vi "Complex Vector.vi"() -> (0 "error out":errorcluster, 3 "Passed?":bool)   [LabVIEW 2009]
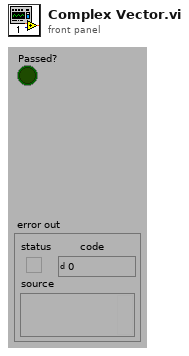
[diagram p1: front panel]
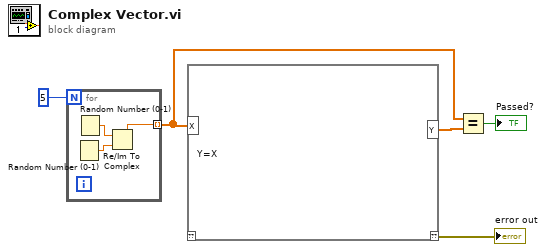
[diagram p0: block diagram]
diagram:
  n1 = for {
    N: 5 -> [_]
    tunnel: [w6] -> w2 mode=indexing
    n2 = Random Number (0-1)() -> (number: 0 to 1=w8:dbl)
    n3 = Random Number (0-1)() -> (number: 0 to 1=w7:dbl)
    n4 = Re/Im To Complex(1:w8, 2:w7) -> (0:w6:cdb)
  }
  n5 = script code="Y=X"("X"=w2) -> ("??"=→"error out":errorcluster, "Y"=w1:cdb[])  [unwired: 1 in]
  n6 = Equal?(x=w2, y=w1) -> (x = y?=→"Passed?":bool)
